vi "KEYNCE_SCANNER.vi"() -> ()   [LabVIEW 2017]
uses:
  Global/DATA LOG.vi
  Global/Global 1.vi
panel:
  out "x+1":i32
  in  "Boolean":bool
  in  "op 60":i32=1
  in  "op 30":i32=2
  in  "op 40":i32=1
  in  "ST 4 STRING 3":string
  in  "ST 3 STRING 2":string
  in  "OP30 ST 2 STRING":string
  out "3":bool
  out "2":bool
  out "1":bool
  in  "Stop Button":bool
  out "SCANNER READ DATA 5":string
  out "SCANNER READ DATA 4":string
  out "SCANNER OP60 DATA":string
  out "SCANNER OP40 DATA":string
  in  "ERROR IN":errorcluster
  out "error out 2":errorcluster
  out "SCANNER OP30 DATA":string
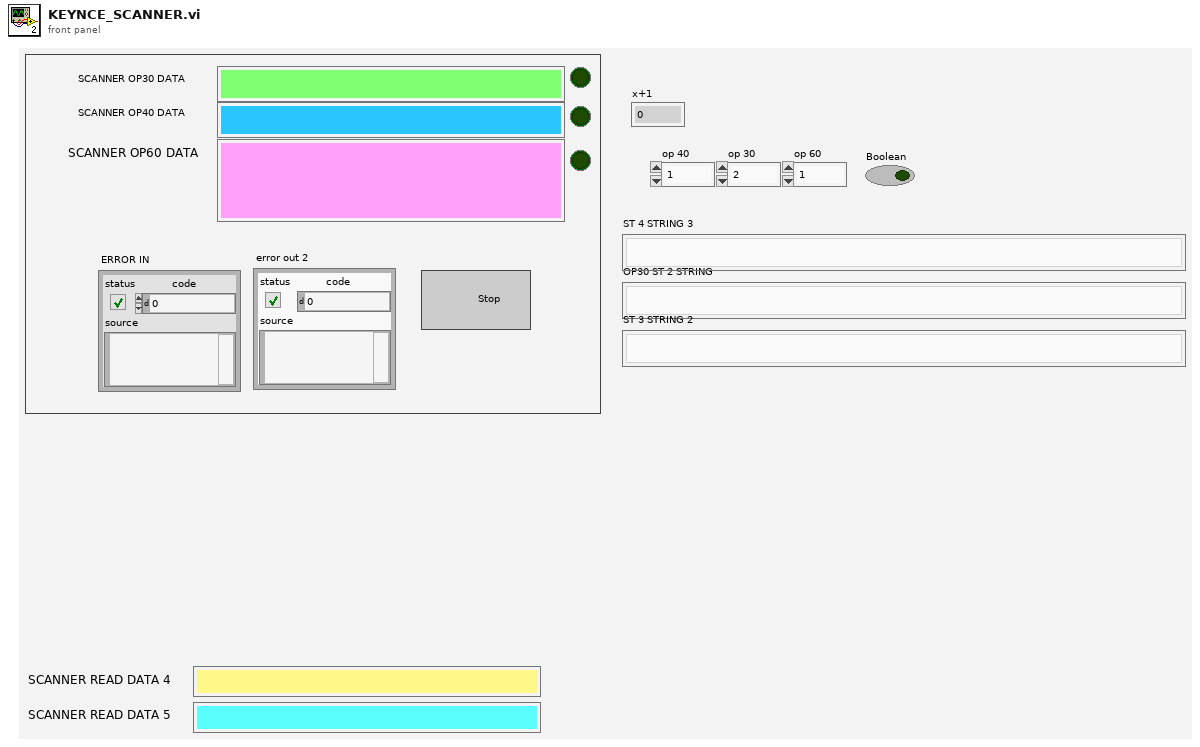
[diagram p1: front panel]
types:
  T1 = enum16{"Standard", "Buffered", "CRLF", "Immediate"}
  T2 = enum32{"invalid app kind", "Development System", "Run Time System", "Student Edition", "Embedded LabVIEW", "Evaluation", "Custom"}
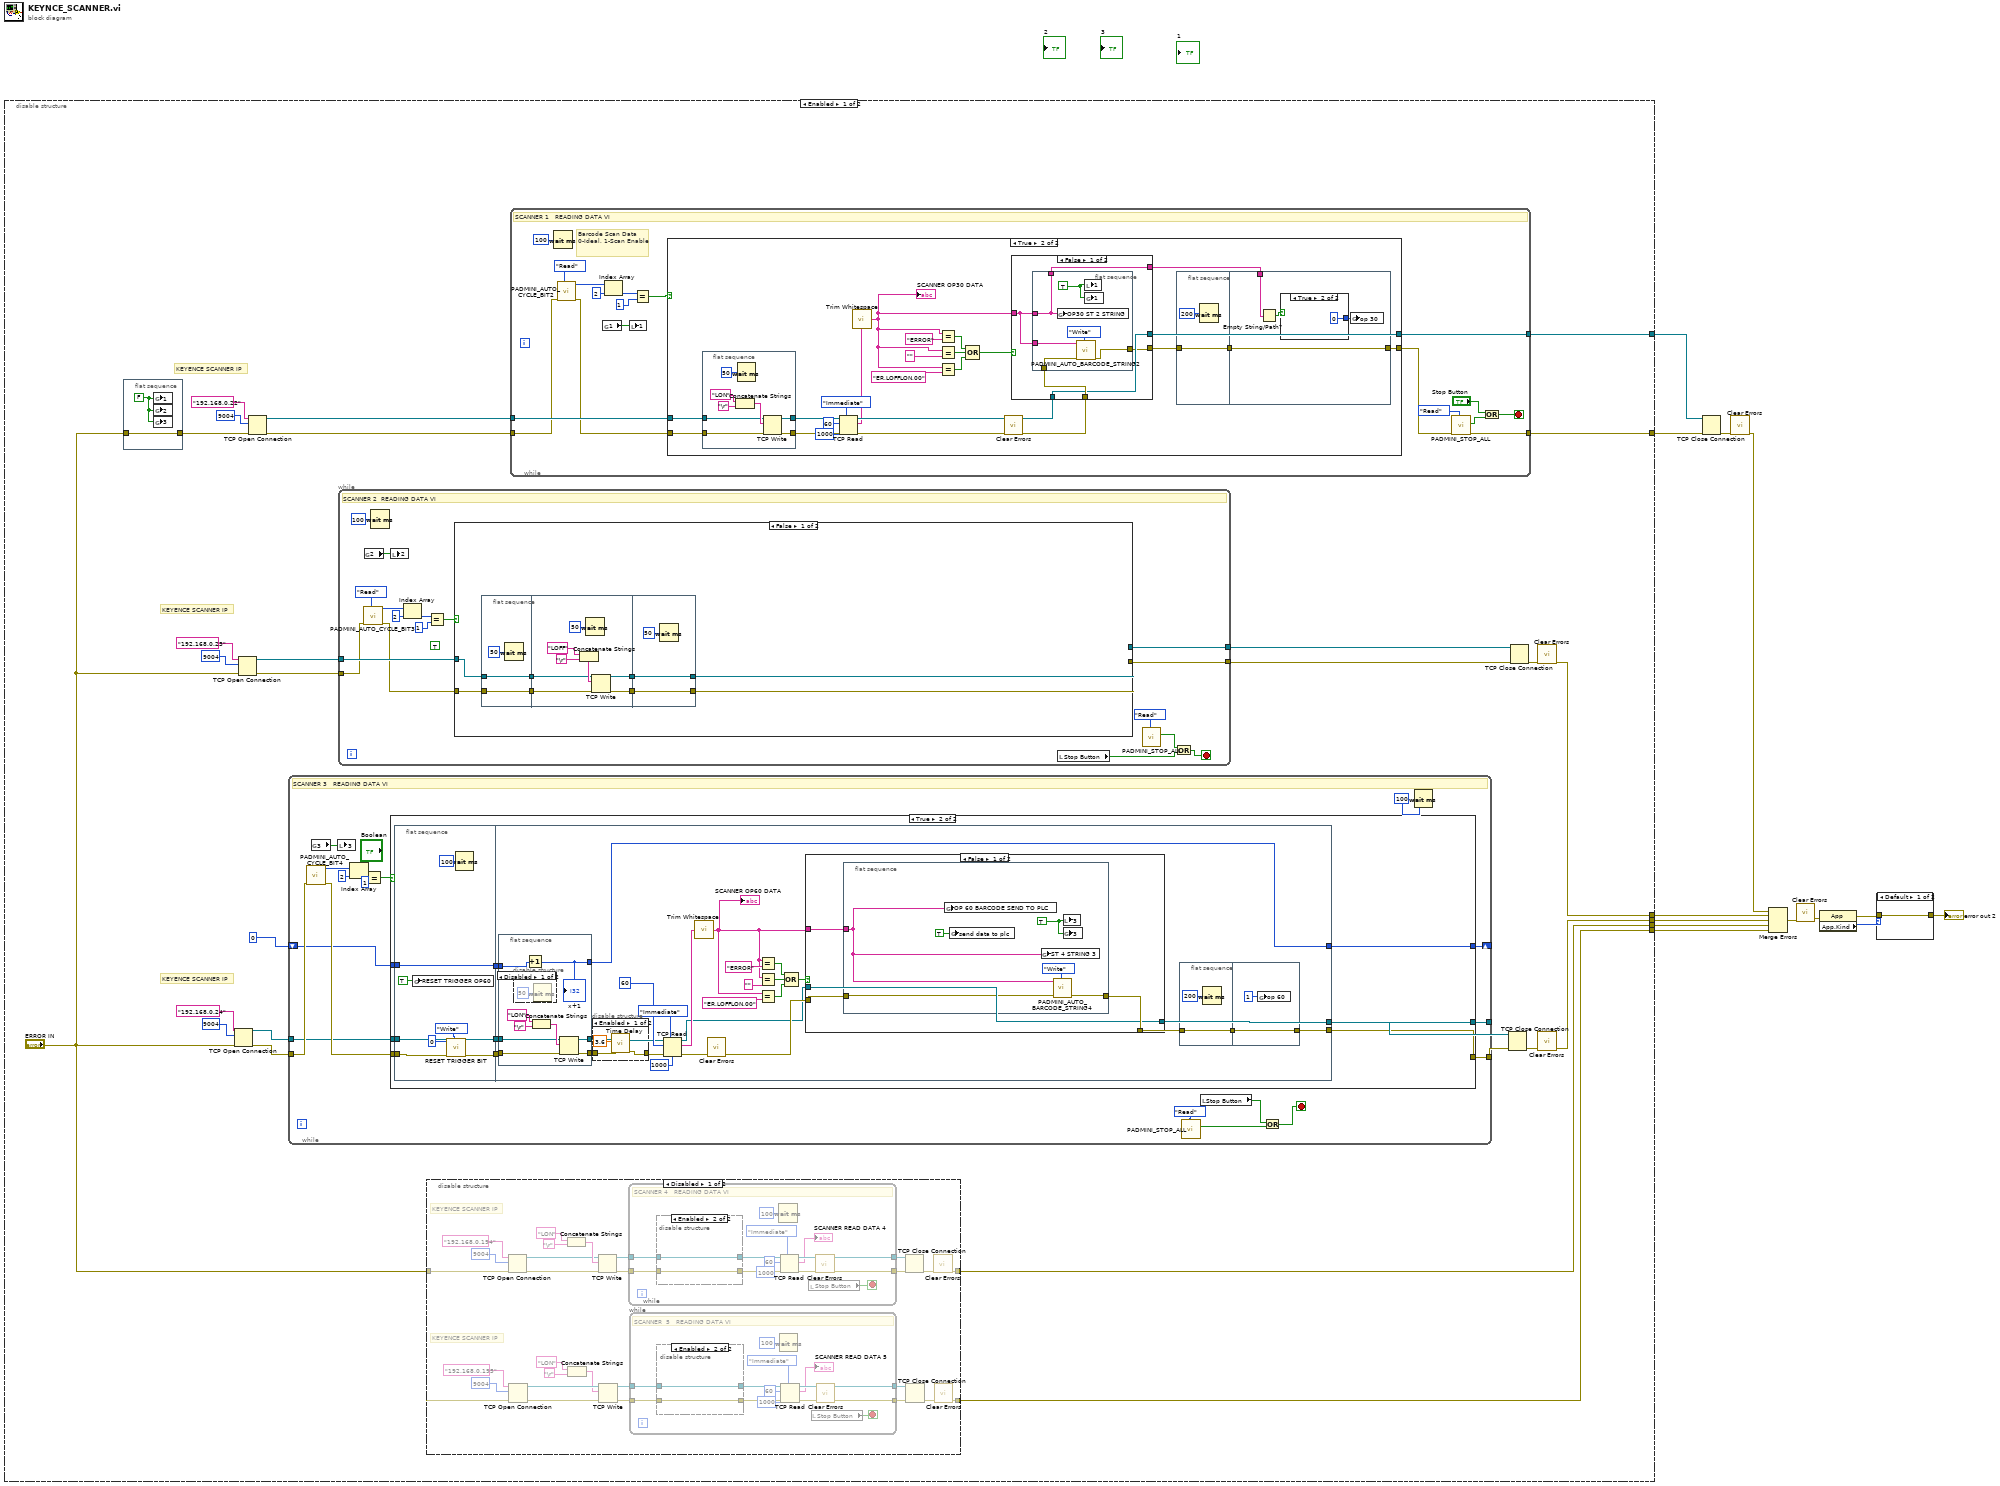
[diagram p0: block diagram]
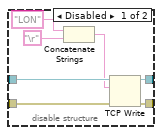
[diagram p2: hidden frame]
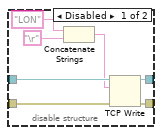
[diagram p3: hidden frame]
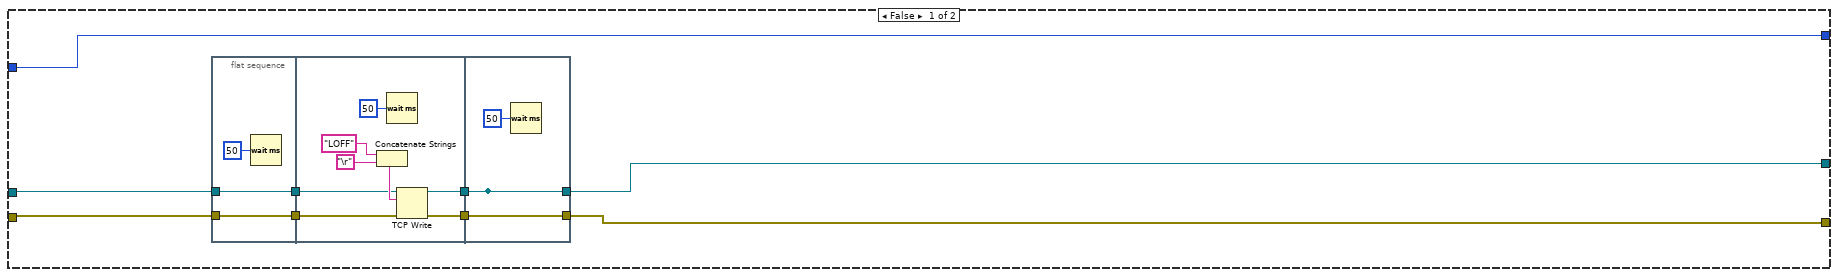
[diagram p5: hidden frame]
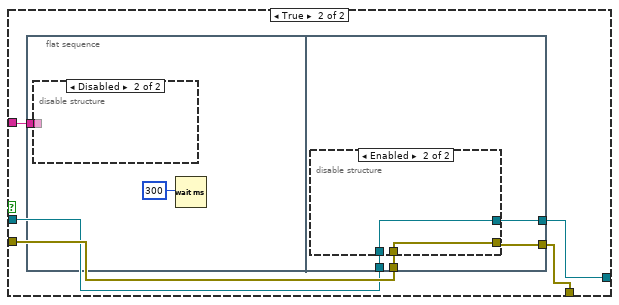
[diagram p8: hidden frame]
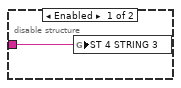
[diagram p9: hidden frame]
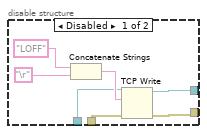
[diagram p10: hidden frame]
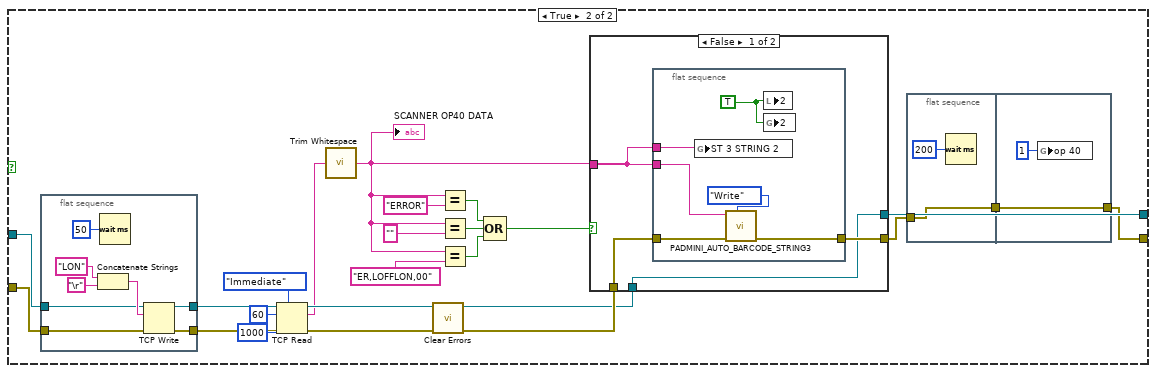
[diagram p11: hidden frame]
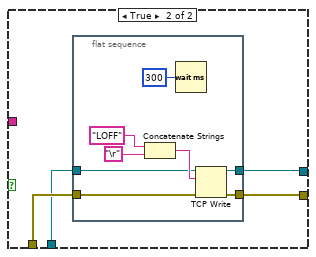
[diagram p12: hidden frame]
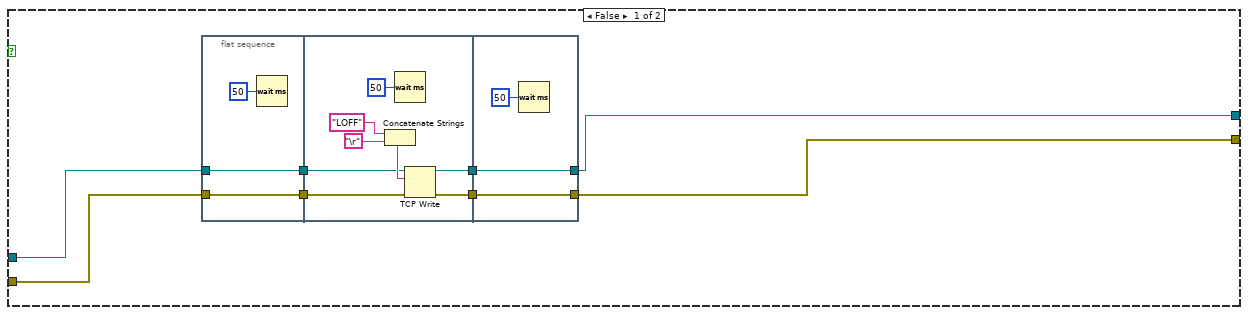
[diagram p13: hidden frame]
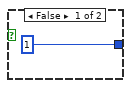
[diagram p14: hidden frame]
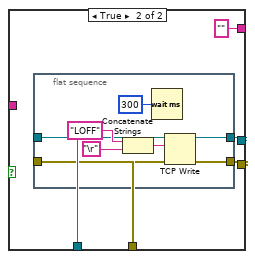
[diagram p15: hidden frame]
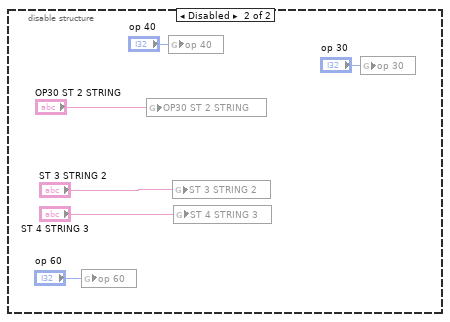
[diagram p16: hidden frame]
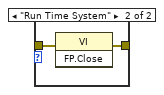
[diagram p17: hidden frame]
diagram:
  n1 = disable-structure shown="Enabled" {
    disable-tunnel: [w34 _] -> w6
    disable-tunnel: [w33 _] -> w5
    disable-tunnel: [w32 _] -> w4
    disable-tunnel: [w31 _] -> w3
    disable-tunnel: [w23 _] -> w2
    disable-tunnel: [w17 _] -> w1
    frame Enabled {
      # "KEYENCE SCANNER IP"
      # "KEYENCE SCANNER IP"
      # "KEYENCE SCANNER IP"
      n2 = flat-sequence {
        tunnel: [w41] -> w15
        tunnel: "ERROR IN" -> [w41]
        frame #0 {
          w42 = FALSE ("1")
          n3 = global write "DATA LOG.vi" "1"(w42) -> ()
          n4 = global write "DATA LOG.vi" "2"(w42) -> ()
          n5 = global write "DATA LOG.vi" "3"(w42) -> ()
        }
      }
      n6 = TCP Open Connection(address="192.168.0.24", remote port or service name=u16 9004, error in (no error)="ERROR IN") -> (connection ID=w29:refnum<k5>, error out=w28:errorcluster)  [unwired: 2 in]
      n7 = TCP Open Connection(address="192.168.0.23", remote port or service name=u16 9004, error in (no error)="ERROR IN") -> (connection ID=w35:refnum<k5>, error out=w36:errorcluster)  [unwired: 2 in]
      n8 = TCP Open Connection(address="192.168.0.22", remote port or service name=u16 9004, error in (no error)=w15) -> (connection ID=w19:refnum<k5>, error out=w18:errorcluster)  [unwired: 2 in]
      n9 = while {
        tunnel: w29 -> [w124]
        tunnel: w28 -> [w130]
        tunnel: [w131] -> w24
        tunnel: [w132] -> w25
        shift-right: [w117] -> _
        shift-left: 0 -> [w118]
        stop <- w119 stop-if-true
        # "SCANNER 3   READING DATA VI"
        n10 = call "PADMINI_AUTO_CYCLE_BIT4.vi"("error in (no error)"=w130) -> ("error out"=w125:errorcluster, "Input 2"=w126:u16[])  [unwired: 9 in]
        n11 = global read "DATA LOG.vi" "3"() -> (w123:bool)
        n12 = local write "3"(w123) -> ()
        n13 = Index Array(array=w126, index=2) -> (element=w127:u16)
        n14 = Equal?(x=w127, y=u16 1) -> (x = y?=w115:bool)
        n15 = case shown="True" w115 {
          tunnel: [w134 w162] -> w132
          tunnel: [w135 w161] -> w131
          tunnel: w125 -> [w137 w164]
          tunnel: w124 -> [w136 w163]
          tunnel: w118 -> [w133 w157]
          tunnel: [w133 w156] -> w117
          frame False {
            n16 = flat-sequence {
              tunnel: w137 -> [w144]
              tunnel: [w144] -> w141
              tunnel: [w142] -> w140
              tunnel: w136 -> [w142]
              tunnel: w141 -> [w149]
              tunnel: [w148] -> w139
              tunnel: [w147] -> w138
              tunnel: w140 -> [w145]
              tunnel: [w153] -> _
              tunnel: [w155] -> w135
              tunnel: w139 -> [w155]
              tunnel: w138 -> [w153]
              tunnel: [w153] -> w134
              frame #0 {
                n17 = Wait (ms)(milliseconds to wait=u32 50) -> ()  [unwired: 1 out]
              }
              frame #1 {
                n18 = Concatenate Strings("LOFF" ("data in"), "\r") -> (w150:string)
                n19 = Wait (ms)(milliseconds to wait=u32 50) -> ()  [unwired: 1 out]
                n20 = TCP Write(connection ID=w145, data in=w150, error in (no error)=w149) -> (connection ID out=w147:refnum<k5>, error out=w148:errorcluster)  [unwired: 1 in, 1 out]
              }
              frame #2 {
                n21 = Wait (ms)(milliseconds to wait=u32 50) -> ()  [unwired: 1 out]
              }
            }
          }
          frame True {
            n22 = flat-sequence {
              tunnel: w163 -> [w172]
              tunnel: w164 -> [w168]
              tunnel: [w167] -> w160
              tunnel: [w172] -> w159
              tunnel: [w170] -> w158
              tunnel: w157 -> [w170]
              tunnel: w160 -> [w192]
              tunnel: w159 -> [w191]
              tunnel: w158 -> [w174]
              tunnel: [w179] -> w162
              tunnel: [w177] -> w161
              tunnel: [w173] -> w156
              frame #0 {
                n23 = global write "Global 1.vi" "RESET TRIGGER OP60"(TRUE ("RESET TRIGGER OP60")) -> ()
                n24 = call "RESET TRIGGER BIT.vi"("Enum"=enum16{"Read", "Write"}."Write", "error in (no error)"=w168, "Numeric"=u16 0) -> ("error out"=w167:errorcluster)  [unwired: 7 in, 1 out]
                n25 = Wait (ms)(milliseconds to wait=u32 100) -> ()  [unwired: 1 out]
              }
              frame #1 {
                n26 = flat-sequence {
                  tunnel: [w212] -> w176
                  tunnel: w192 -> [w213]
                  tunnel: [w210] -> w190
                  tunnel: w191 -> [w211]
                  tunnel: w174 -> [w208]
                  tunnel: [w207] -> w173
                  frame #0 {
                    n27 = disable-structure shown="Disabled" {
                      frame Disabled {
                        n28 = Wait (ms)(milliseconds to wait=u32 50) -> ()  [unwired: 1 out]
                      }
                      frame Enabled {
                      }
                    }
                    n29 = Increment(x=w208) -> (x+1=w207:i32)
                    "x+1" <- w207
                    n30 = Concatenate Strings("LON" ("data in"), "\r") -> (w214:string)
                    n31 = TCP Write(connection ID=w211, data in=w214, error in (no error)=w213) -> (connection ID out=w210:refnum<k5>, error out=w212:errorcluster)  [unwired: 1 in, 1 out]
                  }
                }
                n32 = disable-structure shown="Enabled" {
                  disable-tunnel: w176 -> [w201 w202]
                  disable-tunnel: [w200 w202] -> w175
                  frame Enabled {
                    n33 = call "Time Delay"("error in (no error)"=w201, "Delay Time (s)"=3.6) -> ("error out"=w200:errorcluster)  [unwired: 9 in]
                  }
                  frame Disabled {
                  }
                }
                n34 = TCP Read(connection ID=w190, bytes to read=60, error in (no error)=w175, 7:T1."Immediate" ("mode (standard)"), 9:1000 ("timeout ms (25000)")) -> (connection ID out=w180:refnum<k5>, data out=w184:string, error out=w196:errorcluster)
                n35 = call <vilib>:"Trim Whitespace.vi"("string"=w184) -> ("trimmed string"=w183:string)  [unwired: 1 in]
                "SCANNER OP60 DATA" <- w183
                n36 = call <vilib>:"Clear Errors.vi"("error in (no error)"=w196) -> ("error out"=w193:errorcluster)  [unwired: 5 in, 1 out]
                n37 = Equal?(x=w183, y="ERROR") -> (x = y?=w187:bool)
                n38 = Equal?(x=w183, y="") -> (x = y?=w188:bool)
                n39 = Equal?(x=w183, y="ER,LOFFLON,00") -> (x = y?=w185:bool)
                n40 = Compound Arithmetic op=OR(w187, w188, w185) -> (w181:bool)
                n41 = case shown="False" w181 {
                  tunnel: w193 -> [w220 w229]
                  tunnel: [w219 w231] -> w178
                  tunnel: w183 -> [w218 w227]
                  tunnel: w180 -> [w217 w228]
                  tunnel: [w217 w230] -> w179
                  frame False {
                    n42 = flat-sequence {
                      tunnel: [w224] -> w219
                      tunnel: w220 -> [w225]
                      tunnel: w218 -> [w222]
                      frame #0 {
                        w223 = TRUE ("1")
                        n43 = global write "Global 1.vi" "OP 60 BARCODE SEND TO PLC"(w222) -> ()
                        n44 = global write "Global 1.vi" "send data to plc"(TRUE ("send data to plc")) -> ()
                        n45 = global write "DATA LOG.vi" "ST 4 STRING 3"(w222) -> ()
                        n46 = call "PADMINI_AUTO_BARCODE_STRING4.vi"("Enum"=enum16{"Read", "Write"}."Write", "error in (no error)"=w225, "Input"=w222) -> ("error out"=w224:errorcluster)  [unwired: 7 in, 1 out]
                        n47 = local write "3"(w223) -> ()
                        n48 = global write "DATA LOG.vi" "3"(w223) -> ()
                      }
                    }
                  }
                  frame True {
                    n49 = flat-sequence {
                      tunnel: w227 -> [w232]
                      tunnel: [w235] -> w230
                      tunnel: [w236] -> w231
                      tunnel: w229 -> [w238]
                      tunnel: w228 -> [w237]
                      frame #0 {
                        n50 = disable-structure shown="Disabled" {
                          disable-tunnel: w232 -> [w234 _]
                          frame Enabled {
                            n51 = global write "DATA LOG.vi" "ST 4 STRING 3"(w234) -> ()
                          }
                          frame Disabled {
                          }
                        }
                        n52 = Wait (ms)(milliseconds to wait=u32 300) -> ()  [unwired: 1 out]
                      }
                      frame #1 {
                        n53 = disable-structure shown="Enabled" {
                          disable-tunnel: w238 -> [w242 w246]
                          disable-tunnel: w237 -> [w241 w247]
                          disable-tunnel: [w240 w246] -> w236
                          disable-tunnel: [w239 w247] -> w235
                          frame Disabled {
                            n54 = Concatenate Strings("LOFF" ("data in"), "\r") -> (w245:string)
                            n55 = TCP Write(connection ID=w241, data in=w245, error in (no error)=w242) -> (connection ID out=w239:refnum<k5>, error out=w240:errorcluster)  [unwired: 1 in, 1 out]
                          }
                          frame Enabled {
                          }
                        }
                      }
                    }
                  }
                }
                n56 = flat-sequence {
                  tunnel: w178 -> [w204]
                  tunnel: [w204] -> w198
                  tunnel: [w206] -> w177
                  tunnel: w198 -> [w206]
                  frame #0 {
                    n57 = Wait (ms)(milliseconds to wait=u32 200) -> ()  [unwired: 1 out]
                  }
                  frame #1 {
                    n58 = global write "DATA LOG.vi" "op 60"(1 ("op 30")) -> ()
                  }
                }
              }
            }
          }
        }
        n59 = call "PADMINI_STOP_ALL.vi"("Enum"=enum16{"Read", "Write"}."Read") -> ("Boolean 2"=w121:bool)  [unwired: 9 in, 1 out]
        n60 = local read "Stop Button"() -> (w120:bool)
        n61 = Or(x=w120, y=w121) -> (x .or. y?=w119:bool)
        n62 = Wait (ms)(milliseconds to wait=u32 100) -> ()  [unwired: 1 out]
      }
      n63 = while {
        tunnel: w35 -> [w264]
        tunnel: w36 -> [w261]
        tunnel: [w248] -> w22
        tunnel: [w262] -> w20
        stop <- w249 stop-if-true
        (unwired) TRUE
        # "SCANNER 2  READING DATA VI"
        n64 = call "PADMINI_AUTO_CYCLE_BIT3.vi"("Enum"=enum16{"Read", "Write"}."Read", "error in (no error)"=w261) -> ("error out"=w260:errorcluster, "Input 2"=w255:u16[])  [unwired: 8 in]
        n65 = global read "DATA LOG.vi" "2"() -> (w254:bool)
        n66 = Wait (ms)(milliseconds to wait=u32 100) -> ()  [unwired: 1 out]
        n67 = local write "2"(w254) -> ()
        n68 = Index Array(array=w255, index=2) -> (element=w256:u16)
        n69 = Equal?(x=w256, y=u16 1) -> (x = y?=w253:bool)
        n70 = case shown="False" w253 {
          tunnel: w264 -> [w267 w300]
          tunnel: [w266 w287] -> w248
          tunnel: [w265 w303] -> w262
          tunnel: w260 -> [w269 w302]
          frame False {
            n71 = flat-sequence {
              tunnel: w269 -> [w275]
              tunnel: [w275] -> w272
              tunnel: [w273] -> w268
              tunnel: w267 -> [w273]
              tunnel: w272 -> [w280]
              tunnel: [w279] -> w271
              tunnel: [w278] -> w270
              tunnel: w268 -> [w276]
              tunnel: [w285] -> w265
              tunnel: [w286] -> w266
              tunnel: w271 -> [w286]
              tunnel: w270 -> [w285]
              frame #0 {
                n72 = Wait (ms)(milliseconds to wait=u32 50) -> ()  [unwired: 1 out]
              }
              frame #1 {
                n73 = Concatenate Strings("LOFF" ("data in"), "\r") -> (w281:string)
                n74 = Wait (ms)(milliseconds to wait=u32 50) -> ()  [unwired: 1 out]
                n75 = TCP Write(connection ID=w276, data in=w281, error in (no error)=w280) -> (connection ID out=w278:refnum<k5>, error out=w279:errorcluster)  [unwired: 1 in, 1 out]
              }
              frame #2 {
                n76 = Wait (ms)(milliseconds to wait=u32 50) -> ()  [unwired: 1 out]
              }
            }
          }
          frame True {
            n77 = flat-sequence {
              tunnel: [w318] -> w301
              tunnel: w302 -> [w319]
              tunnel: [w316] -> w299
              tunnel: w300 -> [w317]
              frame #0 {
                n78 = Concatenate Strings("LON" ("data in"), "\r") -> (w320:string)
                n79 = Wait (ms)(milliseconds to wait=u32 50) -> ()  [unwired: 1 out]
                n80 = TCP Write(connection ID=w317, data in=w320, error in (no error)=w319) -> (connection ID out=w316:refnum<k5>, error out=w318:errorcluster)  [unwired: 1 in, 1 out]
              }
            }
            n81 = TCP Read(connection ID=w299, bytes to read=60, error in (no error)=w301, 7:T1."Immediate" ("mode (standard)"), 9:1000 ("timeout ms (25000)")) -> (connection ID out=w304:refnum<k5>, data out=w292:string, error out=w308:errorcluster)
            n82 = call <vilib>:"Trim Whitespace.vi"("string"=w292) -> ("trimmed string"=w290:string)  [unwired: 1 in]
            "SCANNER OP40 DATA" <- w290
            n83 = call <vilib>:"Clear Errors.vi"("error in (no error)"=w308) -> ("error out"=w305:errorcluster)  [unwired: 5 in, 1 out]
            n84 = Equal?(x=w290, y="ERROR") -> (x = y?=w295:bool)
            n85 = Equal?(x=w290, y="") -> (x = y?=w296:bool)
            n86 = Equal?(x=w290, y="ER,LOFFLON,00") -> (x = y?=w293:bool)
            n87 = Compound Arithmetic op=OR(w295, w296, w293) -> (w291:bool)
            n88 = case shown="False" w291 {
              tunnel: w305 -> [w325 w335]
              tunnel: [w324 w333] -> w288
              tunnel: w290 -> [w323 _]
              tunnel: w304 -> [w322 w334]
              tunnel: [w322 w332] -> w303
              frame False {
                n89 = flat-sequence {
                  tunnel: w325 -> [w330]
                  tunnel: w323 -> [w328]
                  tunnel: w323 -> [w327]
                  tunnel: [w329] -> w324
                  frame #0 {
                    w326 = TRUE ("1")
                    n90 = global write "DATA LOG.vi" "ST 3 STRING 2"(w328) -> ()
                    n91 = call "PADMINI_AUTO_BARCODE_STRING3.vi"("Enum"=enum16{"Read", "Write"}."Write", "error in (no error)"=w330, "Input"=w327) -> ("error out"=w329:errorcluster)  [unwired: 7 in, 1 out]
                    n92 = local write "2"(w326) -> ()
                    n93 = global write "DATA LOG.vi" "2"(w326) -> ()
                  }
                }
              }
              frame True {
                n94 = flat-sequence {
                  tunnel: [w340] -> w333
                  tunnel: w335 -> [w341]
                  tunnel: [w338] -> w332
                  tunnel: w334 -> [w339]
                  frame #0 {
                    n95 = Concatenate Strings("LOFF" ("data in"), "\r") -> (w342:string)
                    n96 = Wait (ms)(milliseconds to wait=u32 300) -> ()  [unwired: 1 out]
                    n97 = TCP Write(connection ID=w339, data in=w342, error in (no error)=w341) -> (connection ID out=w338:refnum<k5>, error out=w340:errorcluster)  [unwired: 1 in, 1 out]
                  }
                }
              }
            }
            n98 = flat-sequence {
              tunnel: [w310] -> w289
              tunnel: w288 -> [w310]
              tunnel: [w313] -> w287
              tunnel: w289 -> [w313]
              frame #0 {
                n99 = Wait (ms)(milliseconds to wait=u32 200) -> ()  [unwired: 1 out]
              }
              frame #1 {
                n100 = global write "DATA LOG.vi" "op 40"(1 ("op 30")) -> ()
              }
            }
          }
        }
        n101 = local read "Stop Button"() -> (w250:bool)
        n102 = call "PADMINI_STOP_ALL.vi"("Enum"=enum16{"Read", "Write"}."Read") -> ("Boolean 2"=w251:bool)  [unwired: 9 in, 1 out]
        n103 = Or(x=w251, y=w250) -> (x .or. y?=w249:bool)
      }
      n104 = disable-structure shown="Disabled" {
        disable-tunnel: "ERROR IN" -> [w69 w114]
        disable-tunnel: [w68 w114] -> w32
        disable-tunnel: [w67 w114] -> w31
        frame Disabled {
          # "KEYENCE SCANNER IP"
          # "KEYENCE SCANNER IP"
          n105 = TCP Open Connection(address="192.168.0.194", remote port or service name=u16 9004, error in (no error)=w69) -> (connection ID=w59:refnum<k5>, error out=w61:errorcluster)  [unwired: 2 in]
          n106 = TCP Open Connection(address="192.168.0.195", remote port or service name=u16 9004, error in (no error)=w69) -> (connection ID=w50:refnum<k5>, error out=w48:errorcluster)  [unwired: 2 in]
          n107 = Concatenate Strings("LON" ("data in"), "\r") -> (w64:string)
          n108 = Concatenate Strings("LON" ("data in"), "\r") -> (w45:string)
          n109 = TCP Write(connection ID=w59, data in=w64, error in (no error)=w61) -> (connection ID out=w58:refnum<k5>, error out=w60:errorcluster)  [unwired: 1 in, 1 out]
          n110 = TCP Write(connection ID=w50, data in=w45, error in (no error)=w48) -> (connection ID out=w51:refnum<k5>, error out=w49:errorcluster)  [unwired: 1 in, 1 out]
          n111 = while {
            tunnel: w58 -> [w102]
            tunnel: w60 -> [w104]
            tunnel: [w97] -> w55
            tunnel: [w95] -> w57
            stop <- w92 stop-if-true
            # "SCANNER 4   READING DATA VI"
            n112 = disable-structure shown="Enabled" {
              disable-tunnel: w104 -> [w111 w112]
              disable-tunnel: [w110 w112] -> w103
              disable-tunnel: w102 -> [w109 w113]
              disable-tunnel: [w108 w113] -> w101
              frame Disabled {
                n113 = Concatenate Strings("LON" ("data in"), "\r") -> (w105:string)
                n114 = TCP Write(connection ID=w109, data in=w105, error in (no error)=w111) -> (connection ID out=w108:refnum<k5>, error out=w110:errorcluster)  [unwired: 1 in, 1 out]
              }
              frame Enabled {
              }
            }
            n115 = Wait (ms)(milliseconds to wait=u32 100) -> ()  [unwired: 1 out]
            n116 = TCP Read(connection ID=w101, bytes to read=60, error in (no error)=w103, 7:T1."Immediate" ("mode (standard)"), 9:1000 ("timeout ms (25000)")) -> (connection ID out=w95:refnum<k5>, data out=→"SCANNER READ DATA 4":string, error out=w98:errorcluster)
            n117 = local read "Stop Button"() -> (w92:bool)
            n118 = call <vilib>:"Clear Errors.vi"("error in (no error)"=w98) -> ("error out"=w97:errorcluster)  [unwired: 5 in, 1 out]
          }
          n119 = while {
            tunnel: w51 -> [w80]
            tunnel: w49 -> [w82]
            tunnel: [w75] -> w54
            tunnel: [w73] -> w52
            stop <- w70 stop-if-true
            # "SCANNER  5   READING DATA VI"
            n120 = disable-structure shown="Enabled" {
              disable-tunnel: w82 -> [w89 w90]
              disable-tunnel: [w88 w90] -> w81
              disable-tunnel: w80 -> [w87 w91]
              disable-tunnel: [w86 w91] -> w79
              frame Disabled {
                n121 = Concatenate Strings("LON" ("data in"), "\r") -> (w83:string)
                n122 = TCP Write(connection ID=w87, data in=w83, error in (no error)=w89) -> (connection ID out=w86:refnum<k5>, error out=w88:errorcluster)  [unwired: 1 in, 1 out]
              }
              frame Enabled {
              }
            }
            n123 = Wait (ms)(milliseconds to wait=u32 100) -> ()  [unwired: 1 out]
            n124 = TCP Read(connection ID=w79, bytes to read=60, error in (no error)=w81, 7:T1."Immediate" ("mode (standard)"), 9:1000 ("timeout ms (25000)")) -> (connection ID out=w73:refnum<k5>, data out=→"SCANNER READ DATA 5":string, error out=w76:errorcluster)
            n125 = local read "Stop Button"() -> (w70:bool)
            n126 = call <vilib>:"Clear Errors.vi"("error in (no error)"=w76) -> ("error out"=w75:errorcluster)  [unwired: 5 in, 1 out]
          }
          n127 = TCP Close Connection(connection ID=w57, error in (no error)=w55) -> (error out=w56:errorcluster)  [unwired: 1 in, 1 out]
          n128 = TCP Close Connection(connection ID=w52, error in (no error)=w54) -> (error out=w53:errorcluster)  [unwired: 1 in, 1 out]
          n129 = call <vilib>:"Clear Errors.vi"("error in (no error)"=w56) -> ("error out"=w68:errorcluster)  [unwired: 5 in, 1 out]
          n130 = call <vilib>:"Clear Errors.vi"("error in (no error)"=w53) -> ("error out"=w67:errorcluster)  [unwired: 5 in, 1 out]
        }
        frame Enabled {
        }
      }
      n131 = while {
        tunnel: w19 -> [w361]
        tunnel: w18 -> [w349]
        tunnel: [w358] -> w23
        tunnel: [w354] -> w17
        stop <- w356 stop-if-true
        # "Barcode Scan Data\n0-Ideal, 1-Scan Enable"
        # "SCANNER 1   READING DATA VI"
        n132 = Wait (ms)(milliseconds to wait=u32 100) -> ()  [unwired: 1 out]
        n133 = call "PADMINI_AUTO_CYCLE_BIT2.vi"("Enum"=enum16{"Read", "Write"}."Read", "error in (no error)"=w349) -> ("error out"=w348:errorcluster, "Input 2"=w346:u16[])  [unwired: 8 in]
        n134 = global read "DATA LOG.vi" "1"() -> (w345:bool)
        n135 = Index Array(array=w346, index=2) -> (element=w344:u16)
        n136 = local write "1"(w345) -> ()
        n137 = Equal?(x=w344, y=u16 1) -> (x = y?=w350:bool)
        n138 = case shown="True" w350 {
          tunnel: w348 -> [w369 w400]
          tunnel: w361 -> [w367 w398]
          tunnel: [w366 w401] -> w354
          tunnel: [w368 w385] -> w353
          frame False {
            n139 = flat-sequence {
              tunnel: w367 -> [w371]
              tunnel: w369 -> [w372]
              tunnel: [w372] -> w365
              tunnel: [w371] -> w364
              tunnel: w365 -> [w377]
              tunnel: w364 -> [w375]
              tunnel: [w376] -> w363
              tunnel: [w374] -> w362
              tunnel: [w382] -> w366
              tunnel: [w383] -> w368
              tunnel: w363 -> [w383]
              tunnel: w362 -> [w382]
              frame #0 {
                n140 = Wait (ms)(milliseconds to wait=u32 50) -> ()  [unwired: 1 out]
              }
              frame #1 {
                n141 = Concatenate Strings("LOFF" ("data in"), "\r") -> (w378:string)
                n142 = Wait (ms)(milliseconds to wait=u32 50) -> ()  [unwired: 1 out]
                n143 = TCP Write(connection ID=w375, data in=w378, error in (no error)=w377) -> (connection ID out=w374:refnum<k5>, error out=w376:errorcluster)  [unwired: 1 in, 1 out]
              }
              frame #2 {
                n144 = Wait (ms)(milliseconds to wait=u32 50) -> ()  [unwired: 1 out]
              }
            }
          }
          frame True {
            n145 = flat-sequence {
              tunnel: [w420] -> w399
              tunnel: w400 -> [w421]
              tunnel: [w418] -> w397
              tunnel: w398 -> [w419]
              frame #0 {
                n146 = Concatenate Strings("LON" ("data in"), "\r") -> (w422:string)
                n147 = Wait (ms)(milliseconds to wait=u32 50) -> ()  [unwired: 1 out]
                n148 = TCP Write(connection ID=w419, data in=w422, error in (no error)=w421) -> (connection ID out=w418:refnum<k5>, error out=w420:errorcluster)  [unwired: 1 in, 1 out]
              }
            }
            n149 = TCP Read(connection ID=w397, bytes to read=60, error in (no error)=w399, 7:T1."Immediate" ("mode (standard)"), 9:1000 ("timeout ms (25000)")) -> (connection ID out=w402:refnum<k5>, data out=w389:string, error out=w406:errorcluster)
            n150 = call <vilib>:"Trim Whitespace.vi"("string"=w389) -> ("trimmed string"=w388:string)  [unwired: 1 in]
            "SCANNER OP30 DATA" <- w388
            n151 = Equal?(x=w388, y="ERROR") -> (x = y?=w393:bool)
            n152 = Equal?(x=w388, y="") -> (x = y?=w394:bool)
            n153 = Equal?(x=w388, y="ER,LOFFLON,00") -> (x = y?=w390:bool)
            n154 = Compound Arithmetic op=OR(w393, w394, w390) -> (w392:bool)
            n155 = call <vilib>:"Clear Errors.vi"("error in (no error)"=w406) -> ("error out"=w403:errorcluster)  [unwired: 5 in, 1 out]
            n156 = case shown="False" w392 {
              tunnel: w403 -> [w428 w438]
              tunnel: w388 -> [w427 _]
              tunnel: w402 -> [w426 w439]
              tunnel: [w425 w436] -> w387
              tunnel: [w426 w437] -> w401
              tunnel: [w424 "" ("trimmed string")] -> w384
              frame False {
                n157 = flat-sequence {
                  tunnel: w428 -> [w433]
                  tunnel: w427 -> [w432]
                  tunnel: w427 -> [w429]
                  tunnel: [w430] -> w425
                  tunnel: [w429] -> w424
                  frame #0 {
                    w431 = TRUE ("1")
                    n158 = global write "DATA LOG.vi" "OP30 ST 2 STRING"(w429) -> ()
                    n159 = call "PADMINI_AUTO_BARCODE_STRING2.vi"("Enum"=enum16{"Read", "Write"}."Write", "error in (no error)"=w433, "Input"=w432) -> ("error out"=w430:errorcluster)  [unwired: 7 in, 1 out]
                    n160 = local write "1"(w431) -> ()
                    n161 = global write "DATA LOG.vi" "1"(w431) -> ()
                  }
                }
              }
              frame True {
                n162 = flat-sequence {
                  tunnel: [w444] -> w436
                  tunnel: w438 -> [w445]
                  tunnel: [w442] -> w437
                  tunnel: w439 -> [w443]
                  frame #0 {
                    n163 = Concatenate Strings("LOFF" ("data in"), "\r") -> (w446:string)
                    n164 = Wait (ms)(milliseconds to wait=u32 300) -> ()  [unwired: 1 out]
                    n165 = TCP Write(connection ID=w443, data in=w446, error in (no error)=w445) -> (connection ID out=w442:refnum<k5>, error out=w444:errorcluster)  [unwired: 1 in, 1 out]
                  }
                }
              }
            }
            n166 = flat-sequence {
              tunnel: w387 -> [w409]
              tunnel: [w409] -> w386
              tunnel: [w413] -> w385
              tunnel: w386 -> [w413]
              tunnel: w384 -> [w411]
              frame #0 {
                n167 = Wait (ms)(milliseconds to wait=u32 200) -> ()  [unwired: 1 out]
              }
              frame #1 {
                n168 = Empty String/Path?(string/path=w411) -> (empty?=w412:bool)
                n169 = case shown="True" w412 {
                  tunnel: [1 ("op 30") 0 ("op 30")] -> w410
                  frame False {
                  }
                  frame True {
                  }
                }
                n170 = global write "DATA LOG.vi" "op 30"(w410) -> ()
              }
            }
          }
        }
        n171 = call "PADMINI_STOP_ALL.vi"("Enum"=enum16{"Read", "Write"}."Read", "error in (no error)"=w353) -> ("error out"=w358:errorcluster, "Boolean 2"=w357:bool)  [unwired: 8 in]
        n172 = Or(x="Stop Button", y=w357) -> (x .or. y?=w356:bool)
      }
      n173 = TCP Close Connection(connection ID=w25, error in (no error)=w24) -> (error out=w30:errorcluster)  [unwired: 1 in, 1 out]
      n174 = TCP Close Connection(connection ID=w20, error in (no error)=w22) -> (error out=w21:errorcluster)  [unwired: 1 in, 1 out]
      n175 = call <vilib>:"Clear Errors.vi"("error in (no error)"=w21) -> ("error out"=w34:errorcluster)  [unwired: 5 in, 1 out]
      n176 = call <vilib>:"Clear Errors.vi"("error in (no error)"=w30) -> ("error out"=w33:errorcluster)  [unwired: 5 in, 1 out]
    }
    frame Disabled {
      n177 = global write "DATA LOG.vi" "op 60"("op 60") -> ()
      n178 = global write "DATA LOG.vi" "OP30 ST 2 STRING"("OP30 ST 2 STRING") -> ()
      n179 = global write "DATA LOG.vi" "op 40"("op 40") -> ()
      n180 = global write "DATA LOG.vi" "ST 3 STRING 2"("ST 3 STRING 2") -> ()
      n181 = global write "DATA LOG.vi" "ST 4 STRING 3"("ST 4 STRING 3") -> ()
      n182 = global write "DATA LOG.vi" "op 30"("op 30") -> ()
    }
  }
  n183 = TCP Close Connection(connection ID=w1, error in (no error)=w2) -> (error out=w7:errorcluster)  [unwired: 1 in, 1 out]
  n184 = call <vilib>:"Clear Errors.vi"("error in (no error)"=w7) -> ("error out"=w9:errorcluster)  [unwired: 5 in, 1 out]
  n185 = Merge Errors(w9, w6, w5, w4, w3) -> (w8:errorcluster)
  n186 = call <vilib>:"Clear Errors.vi"("error in (no error)"=w8) -> ("error out"=w11:errorcluster)  [unwired: 5 in, 1 out]
  n187 = property class="App"(error in=w11) -> (error out=w12:errorcluster, "App.Kind"=w13:T2)  [unwired: 1 in, 1 out]
  n188 = case shown="Default" w13 {
    tunnel: w12 -> [w454 w456]
    tunnel: [w454 w455] -> w10
    frame Default {
    }
    frame "Run Time System" {
      n189 = invoke class="VI" method="FP.Close"(error in=w456) -> (error out=w455:errorcluster)  [unwired: 2 in, 2 out]
    }
  }
  "error out 2" <- w10
